vi "AB_API Set Inclusion.vi"(7 "top tree? (true)":bool, 8 "error in (no error)":errorcluster, 10 "Source in":refnum<class "AB_Source.lvclass">, 11 "Build in":refnum<class "AB_Build.lvclass">) -> (0 "error out":errorcluster, 2 "AB_Source_VI out":refnum<class "AB_Source.lvclass">, 3 "AB_Build out":refnum<class "AB_Build.lvclass">)   [LabVIEW 2020]
uses:
  <vilib>/AppBuilder/AB_Classes/Build/AB_Build.lvclass
  <vilib>/AppBuilder/AB_Classes/Source/AB_Source.lvclass
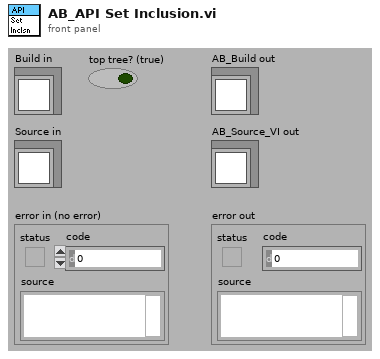
[diagram p1: front panel]
types:
  T1 = typedef "AB_UI_Page_Source_Files_supportedFunctions.ctl" = cluster{"topTreeInclusion":T2, "bottomTreeInclusion":T2}
  T2 = typedef "AB_Source_Inclusion.ctl" = enum16{"IncludeIfReferenced", "Include", "Exclude", "TopLevel"}
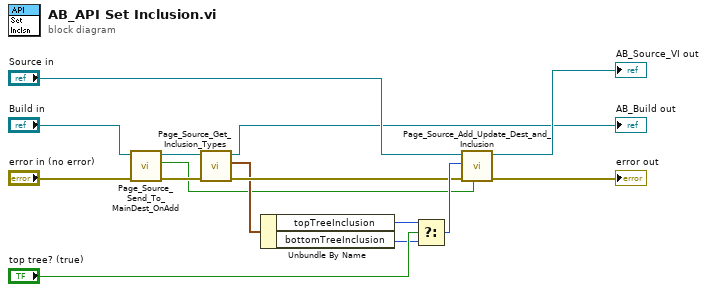
[diagram p0: block diagram]
diagram:
  n1 = call-dynamic "Page_Source_Send_To_MainDest_OnAdd.vi"("error in (no error)"="error in (no error)", "AB_Build in"="Build in") -> ("error out"=w10:errorcluster, "send to main dest"=w7:bool, "AB_Build out"=w8:refnum<class "AB_Build.lvclass">)  [unwired: 7 out]
  n2 = call-dynamic "Page_Source_Get_Inclusion_Types.vi"("error in (no error)"=w10, "AB_Build in"=w8) -> ("error out"=w11:errorcluster, "supportedFunctions"=w9:T1, "AB_Build out"=→"AB_Build out":refnum<class "AB_Build.lvclass">)  [unwired: 7 out]
  n3 = Unbundle By Name(w9) -> ("topTreeInclusion"=w13:T2, "bottomTreeInclusion"=w12:T2)
  n4 = Select(t=w13, s="top tree? (true)", f=w12) -> (s? t:f=w14:T2)
  n5 = call <vilib>:"Page_Source_Add_Update_Dest_and_Inclusion.vi"("send to main destination?"=w7, "error in (no error)"=w11, "Inclusion"=w14, "AB_Source_VI in"="Source in") -> ("error out"=→"error out":errorcluster, "AB_Source_VI out"=→"AB_Source_VI out":refnum<class "AB_Source.lvclass">)  [unwired: 6 out]
